vi "Status Setpoint 2.vi"(5 "Retry Attempts (0)":i32 min=0, 7 "Unit Address (-1)":i32=-1, 8 "error in (no error)":errorcluster, 11 "VISA resource name (in)":refnum<visa-resource-name>) -> (0 "error out":errorcluster, 1 "Setpoint Type":T1, 2 "Setpoint 2":string, 3 "VISA resource name (out)":refnum<visa-resource-name>)   [LabVIEW 2020, in "Omega Platinum Series.lvlib"]
doc: "Get setpoint 2 for the controller."
uses:
  Omega Platinum Series.lvlib
  Type Defs/Setpoint Type.ctl
panel:
  out "Command":string
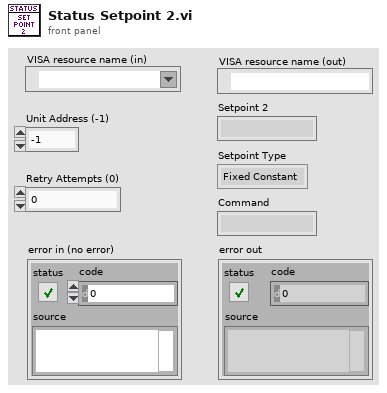
[diagram p1: front panel]
types:
  T1 = typedef "Omega Platinum Series.lvlib/Setpoint Type.ctl" = enum16{"Fixed Constant", "Deviation"}
  T2 = typedef "Omega Platinum Series.lvlib/Response.ctl" = cluster{"Unit Address":i32, "Command Class":string, "Command ID":u32, "Parameters":string}
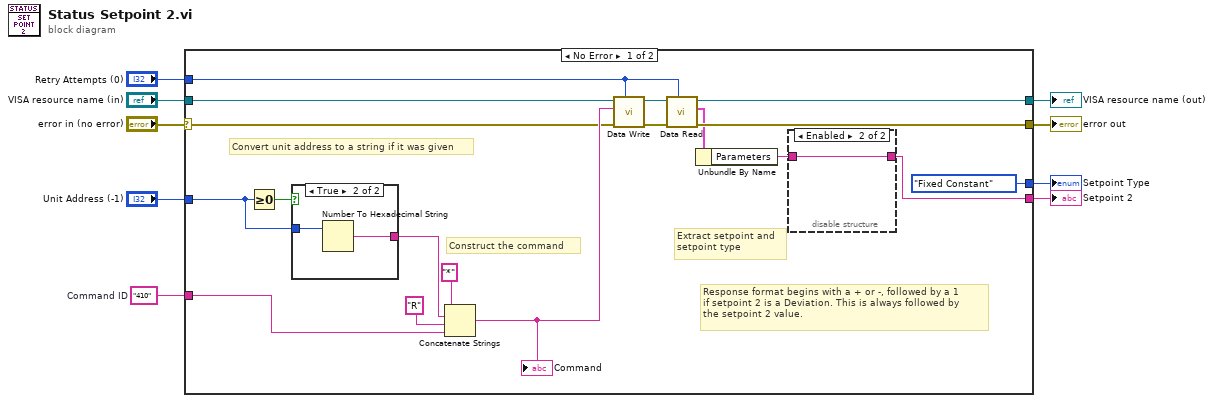
[diagram p0: block diagram]
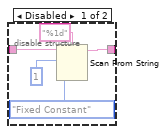
[diagram p2: hidden frame]
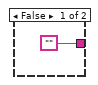
[diagram p3: hidden frame]
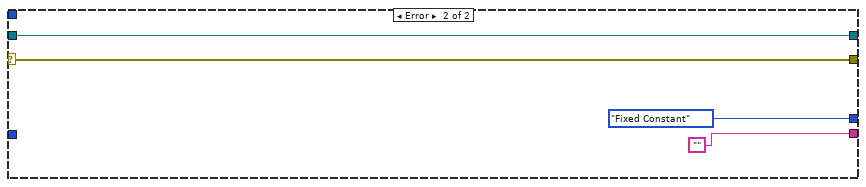
[diagram p4: hidden frame]
diagram:
  w9 = "410"  # Command ID
  n1 = case shown="No Error" "error in (no error)" {
    selector: "error in (no error)" -> [w21 w40]
    tunnel: w9 -> [w15 _]
    tunnel: "Unit Address (-1)" -> [w25 _]
    tunnel: [w17 w40] -> w6
    tunnel: "VISA resource name (in)" -> [w23 w39]
    tunnel: [w18 w39] -> w4
    tunnel: [w12 ""] -> w3
    tunnel: [Setpoint_Type."Fixed Constant" ("Setpoint Type") Setpoint_Type."Fixed Constant" ("Setpoint Type")] -> w2
    tunnel: "Retry Attempts (0)" -> [w10 _]
    frame No Error {
      # "Response format begins with a + or -, followed by a 1 \nif setpoint 2 is a Deviation. This is always followed by\nthe setpoint 2 value."
      # "Extract setpoint and \nsetpoint type"
      # "Convert unit address to a string if it was given"
      # "Construct the command"
      n2 = Greater Or Equal To 0?(x=w25) -> (x >= 0?=w27:bool)
      n3 = case shown="True" w27 {
        tunnel: w25 -> [_ w36]
        tunnel: ["" w35] -> w24
        frame False {
        }
        frame True {
          n4 = Number To Hexadecimal String(2:w36) -> (0:w35:string)  [unwired: 1 in]
        }
      }
      n5 = Concatenate Strings("*" ("string"), w24, "R" ("string"), w15) -> (w22:string)
      "Command" <- w22
      n6 = call "Data Write.vi"("Retry Attempts (0)"=w10, "error in (no error)"=w21, "Command"=w22, "VISA Refnum in"=w23) -> ("error out"=w20:errorcluster, "VISA Refnum out"=w19:refnum<visa-resource-name>)  [unwired: 6 in]
      n7 = call "Data Read.vi"("Retry Attempts (0)"=w10, "error in (no error)"=w20, "VISA Refnum in"=w19) -> ("error out"=w17:errorcluster, "Response Cluster"=w14:T2, "VISA Refnum out"=w18:refnum<visa-resource-name>)  [unwired: 5 in, 1 out]
      n8 = Unbundle By Name(w14) -> ("Parameters"=w13:string)
      n9 = disable-structure shown="Enabled" {
        disable-tunnel: w13 -> [w32 w33]
        disable-tunnel: [w29 w33] -> w12
        frame Disabled {
          n10 = Scan From String(format string="%1d", input string=w32, initial scan location=u32 1, default 1=Setpoint_Type."Fixed Constant" ("Setpoint Type")) -> (remaining string=w29:string)  [unwired: 2 in, 2 out]
        }
        frame Enabled {
        }
      }
    }
    frame Error {
    }
  }
  "error out" <- w6
  "VISA resource name (out)" <- w4
  "Setpoint 2" <- w3
  "Setpoint Type" <- w2
